vi "XY to (x,y).vi"   [LabVIEW 2019, in "xy_utilities.lvlib"]
doc: "Convert <b>XY-data</b> (cluster of arrays of X and Y) to <b>(x,y)</b> coordinates (array of clusters of (x,y) values).\n\nWire data to the data input to determine the polymorphic instance to use or manually select the instance."
uses:
  xy_utilities.lvlib
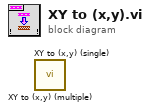
[diagram p0: block diagram]
diagram:
  n1 = call "XY to (x,y) (multiple).vi"() -> ()  [unwired: 9 in, 3 out]
  n2 = call "XY to (x,y) (single).vi"() -> ()  [unwired: 9 in, 3 out]
